vi "Dynamixel MX-Series Decode Pos Data FPGA.vi"(9 "ScaleOutput":fxp<+/-,25,16>=0.349609375, 11 "RecData":u8[](array[numeric])) -> (0 "Error":bool, 1 "Csum":u8, 3 "Position":fxp<+/-,24,16>)   [LabVIEW 2015]
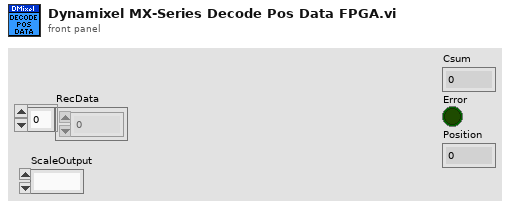
[diagram p1: front panel]
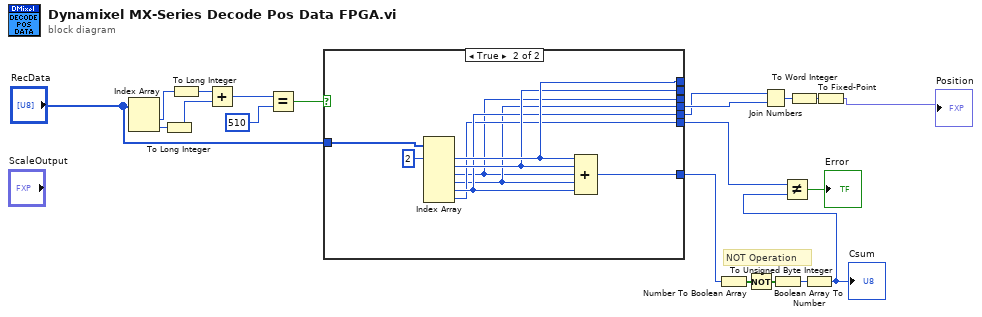
[diagram p0: block diagram]
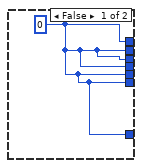
[diagram p2: hidden frame]
diagram:
  # "NOT Operation"
  n1 = Index Array(array="RecData") -> (element #1=w13:u8, element #2=w14:u8)  [unwired: 2 in]
  n2 = To Long Integer(number=w14) -> (32bit integer=w11:i32)
  n3 = To Long Integer(number=w13) -> (32bit integer=w12:i32)
  n4 = Add(x=w12, y=w11) -> (x+y=w10:i32)
  n5 = Equal?(x=w10, y=510) -> (x = y?=w16:bool)
  n6 = case shown="True" w16 {
    tunnel: [w21 w28] -> _
    tunnel: [w21 w26] -> _
    tunnel: [w21 w22] -> _
    tunnel: [w21 w23] -> w5
    tunnel: [w21 w25] -> w4
    tunnel: [w21 w24] -> w9
    tunnel: [w21 w30] -> w15
    tunnel: "RecData" -> [_ w27]
    frame False {
      w21 = u8 0
    }
    frame True {
      n7 = Index Array(array=w27, index #1=2 ("index")) -> (element #1=w28:u8, element #2=w26:u8, element #3=w22:u8, element #4=w23:u8, element #5=w25:u8, element #6=w24:u8)  [unwired: 5 in]
      n8 = Compound Arithmetic op=ADD(w28, w26, w22, w23, w25) -> (w30:u8)
    }
  }
  n9 = Number To Boolean Array(number=w15) -> (Boolean array=w18:bool[])
  n10 = Not(x=w18) -> (.not. x?=w19:bool[])
  n11 = Join Numbers(hi=w4, lo=w5) -> ((hi.lo)=w3:u16)
  n12 = Boolean Array To Number(Boolean array=w19) -> (number=w20:u32)
  n13 = To Word Integer(number=w3) -> (16bit integer=w2:i16)
  n14 = To Unsigned Byte Integer(number=w20) -> (unsigned 8bit integer=w8:u8)
  "Csum" <- w8
  n15 = Not Equal?(x=w9, y=w8) -> (x != y?=→"Error":bool)
  n16 = To Fixed-Point(number=w2) -> (fixed-point=→"Position":fxp<+/-,24,16>)  [unwired: 1 in]
